vi "Data Display Loop.vi"(10 "Data":refnum<vi>, 11 "Notifier in":T1) -> ()   [LabVIEW 2018]
uses:
  library/something else/Controls/Data Notifier.ctl
  library/something else/Controls/Acquired Data.ctl
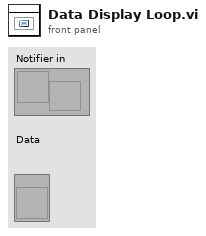
[diagram p1: front panel]
types:
  T1 = typedef "Data Notifier.ctl" = refnum<notifier>
  T2 = typedef "Acquired Data.ctl" = waveform(dbl)[]
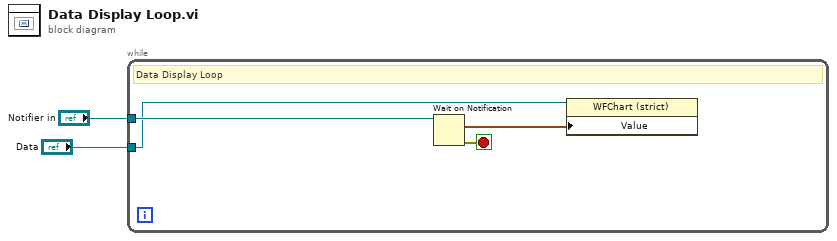
[diagram p0: block diagram]
diagram:
  n1 = while "Data Display Loop" {
    tunnel: "Notifier in" -> [w6]
    tunnel: "Data" -> [w4]
    stop <- w5 stop-if-true
    # "Data Display Loop"
    n2 = Wait on Notification(notifier=w6) -> (notification=w3:T2, error out=w5:errorcluster)  [unwired: 3 in, 2 out]
    n3 = property class="WFChart (strict)"(reference=w4, "Value"=w3) -> ()  [unwired: 1 in, 2 out]
  }
